vi "setSettings.vi"(10 "Settings":T1={"IPAddress"="127.0.0.1", "Port"=0, "StartupScript"="source /usr/ts_sal/setup.env && /usr/ts_sal/test/m1m3/cpp/src/SALPipe %d -1"}, 11 "M1M3SAL in":refnum<class "M1M3SAL.lvclass">) -> (3 "M1M3SAL out":refnum<class "M1M3SAL.lvclass">)   [LabVIEW 2016, in "M1M3Communicator.lvlib" / "M1M3SAL.lvclass"]
uses:
  M1M3SAL.lvclass
  DataTypes/M1M3SALSettings.ctl
  M1M3SAL.lvclass/M1M3SAL.ctl
  M1M3Communicator.lvlib
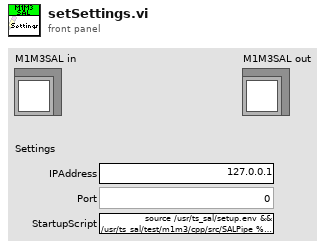
[diagram p1: front panel]
types:
  T1 = typedef "M1M3Communicator.lvlib/M1M3SALSettings.ctl" = cluster{"IPAddress":string, "Port":u16, "StartupScript":string}
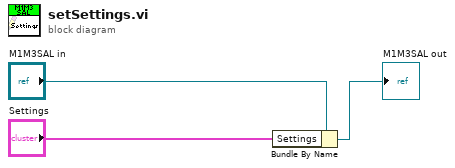
[diagram p0: block diagram]
diagram:
  n1 = Bundle By Name(cluster="M1M3SAL in", "Settings"="Settings") -> (→"M1M3SAL out":refnum<class "M1M3SAL.lvclass">)
